vi "Broadcast Batch Messages.vi"(8 "error in (no error)":errorcluster, 9 "Mail Strategy In":refnum<class "Mail Strategy.lvclass">, 10 "Messages In":refnum<class "Message.lvclass">[](array[class]), 11 "Simple Map Queue Group Messenger in":refnum<class "Simple Map Queue Group Messenger.lvclass">) -> (0 "error out":errorcluster, 3 "Simple Map Queue Group Messenger out":refnum<class "Simple Map Queue Group Messenger.lvclass">)   [LabVIEW 2024, in "Simple Map Queue Group Messenger.lvclass"]
uses:
  Simple Map Queue Group Messenger.lvclass
  Ancestor Class/Message/Message.lvclass
  Ancestor Class/Messenger/Mail Strategy/Mail Strategy.lvclass
  Simple Map Queue Group Messenger.lvclass/Simple Map Queue Group Messenger.ctl
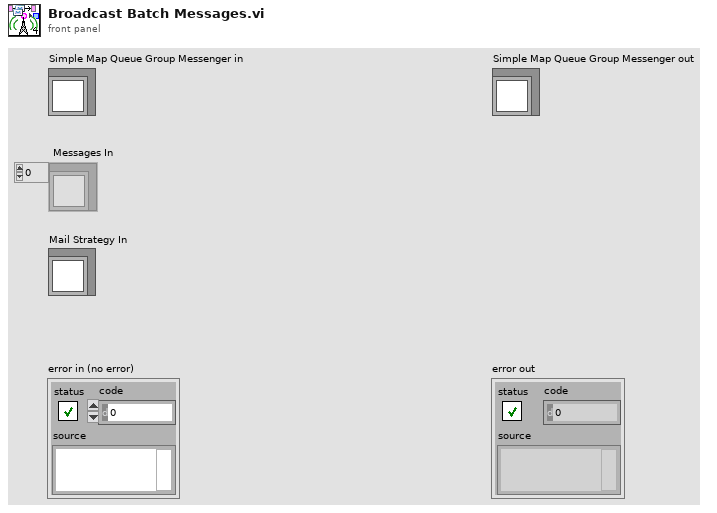
[diagram p1: front panel]
types:
  T1 = typedef "Queue Group Map.ctl" = map{i64, T2[]}
  T2 = typedef "Message Queue.ctl" = refnum<queue>
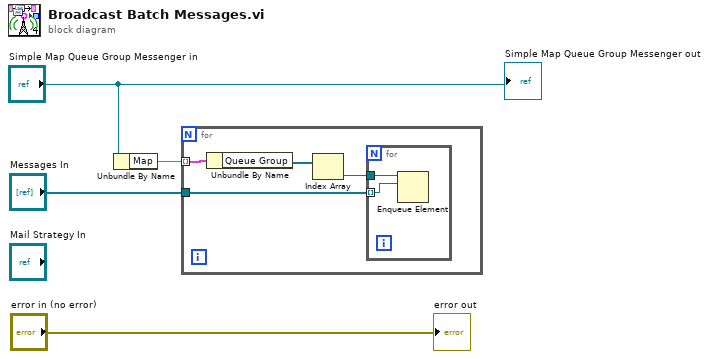
[diagram p0: block diagram]
diagram:
  n1 = Unbundle By Name("Simple Map Queue Group Messenger in") -> ("Map"=w2:T1)
  n2 = for {
    tunnel: w2 -> [w8] mode=indexing
    tunnel: "Messages In" -> [w5]
    n3 = Unbundle By Name(w8) -> ("Queue Group"=w7:T2[])
    n4 = Index Array(array=w7) -> (element=w6:T2)  [unwired: 1 in]
    n5 = for {
      tunnel: w6 -> [w10]
      tunnel: w5 -> [w9] mode=indexing
      n6 = Enqueue Element(queue=w10, element=w9) -> ()  [unwired: 2 in, 3 out]
    }
  }
  "error out" <- "error in (no error)"
  "Simple Map Queue Group Messenger out" <- "Simple Map Queue Group Messenger in"
